vi "isRootEmbbedService.vi"(11 "device":string) -> (2 "detail":string, 3 "type":u16)   [LabVIEW 2010]
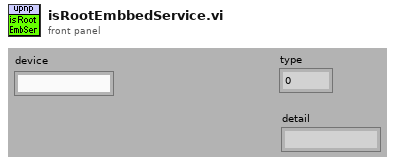
[diagram p1: front panel]
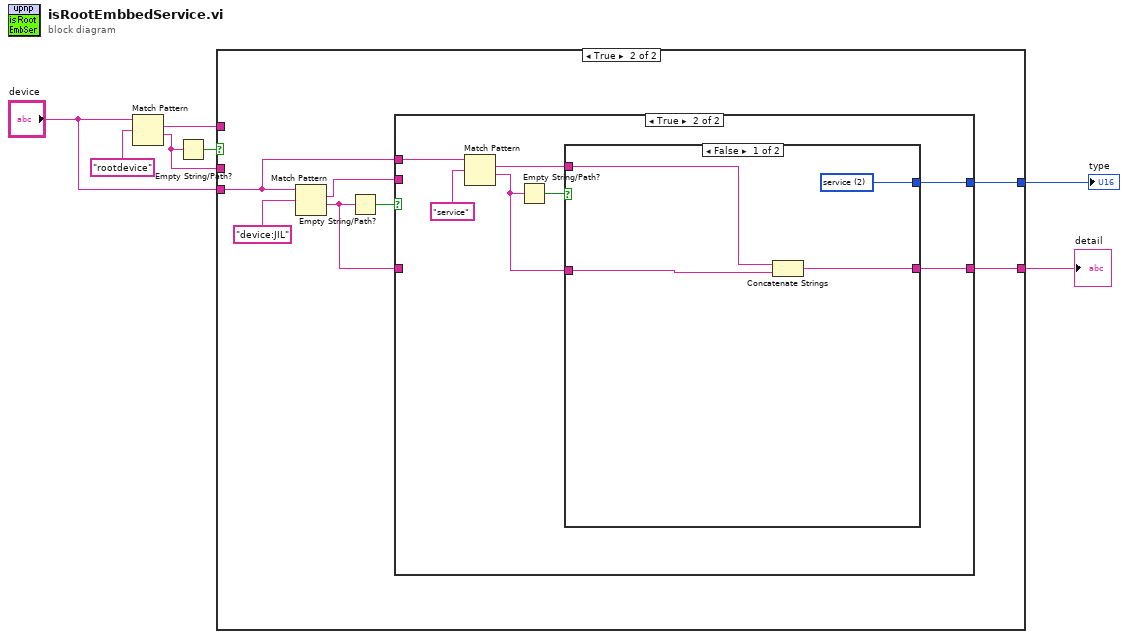
[diagram p0: block diagram]
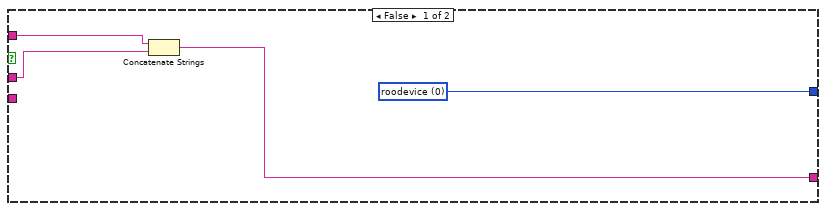
[diagram p2: hidden frame]
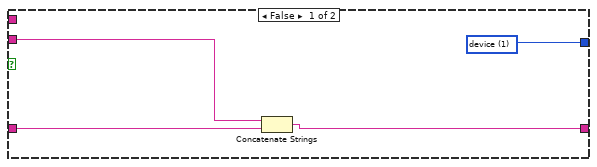
[diagram p3: hidden frame]
diagram:
  n1 = Match Pattern(string="device", regular expression="rootdevice") -> (match substring=w1:string, after substring=w2:string)  [unwired: 3 out]
  n2 = Empty String/Path?(string/path=w2) -> (empty?=w6:bool)
  n3 = case shown="True" w6 {
    tunnel: "device" -> [_ w16]
    tunnel: [w11 w15] -> w4
    tunnel: [w8 w14] -> w3
    tunnel: w2 -> [w9 _]
    tunnel: w1 -> [w10 _]
    frame False {
      w11 = u16 0 items=["roodevice", "device", "service"] ("Ring")
      n4 = Concatenate Strings(w10, w9) -> (w8:string)
    }
    frame True {
      n5 = Match Pattern(string=w16, regular expression="device:JIL") -> (match substring=w12:string, after substring=w13:string)  [unwired: 3 out]
      n6 = Empty String/Path?(string/path=w13) -> (empty?=w17:bool)
      n7 = case shown="True" w17 {
        tunnel: w16 -> [_ w28]
        tunnel: [w22 w26] -> w15
        tunnel: [w19 w24] -> w14
        tunnel: w13 -> [w20 _]
        tunnel: w12 -> [w21 _]
        frame False {
          w22 = u16 1 items=["roodevice", "device", "service"] ("Ring")
          n8 = Concatenate Strings(w21, w20) -> (w19:string)
        }
        frame True {
          n9 = Match Pattern(string=w28, regular expression="service") -> (match substring=w23:string, after substring=w25:string)  [unwired: 3 out]
          n10 = Empty String/Path?(string/path=w25) -> (empty?=w27:bool)
          n11 = case shown="False" w27 {
            tunnel: [w33 _] -> w26
            tunnel: [w30 w34] -> w24
            tunnel: w25 -> [w31 w34]
            tunnel: w23 -> [w32 _]
            frame False {
              w33 = u16 2 items=["roodevice", "device", "service"] ("Ring")
              n12 = Concatenate Strings(w32, w31) -> (w30:string)
            }
            frame True {
            }
          }
        }
      }
    }
  }
  "type" <- w4
  "detail" <- w3
